vi "FPGARPM.vi"() -> (1 "RPM1 Period (ms)":u32)   [LabVIEW 2019]
uses:
  <vilib>/rvi/Emulation/niFpgaGetClockAttributes.vi
  <vilib>/rvi/Emulation/niFpgaSctlEmulationGetInTimedLoop.vi
  <vilib>/rvi/Emulation/niFpgaEmulationReportErrorSimple.vi
  <vilib>/rvi/eio/common/nirviEmuTemplateMethod_errors.vi
  <vilib>/rvi/Emulation/niFpgaCriticalErrorInLSC.vi
  <vilib>/eio/EIONode/EIONode.xnode
panel:
  out "RPM2 Period (ms)":i16
  # "READ Rotational Speed"
  # "AM Series Inductive Proximity Sensors"
  # "AM1-A0-4H"
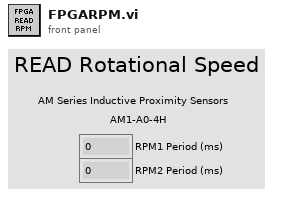
[diagram p1: front panel]
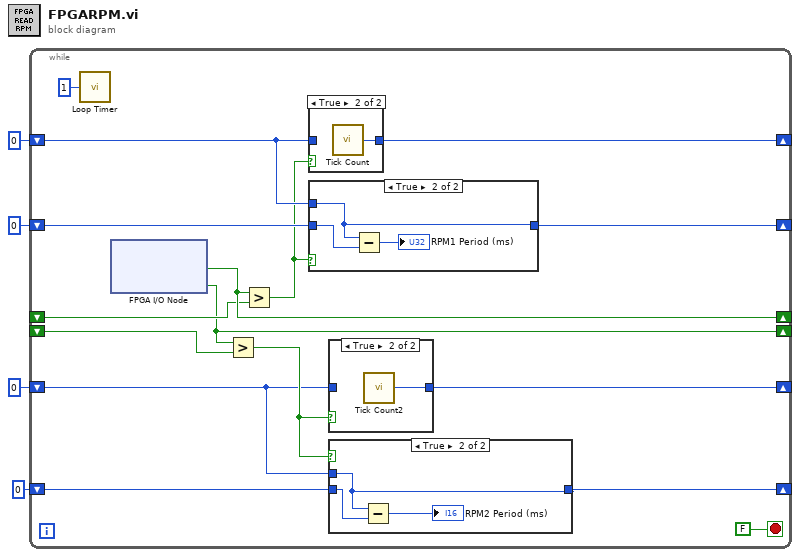
[diagram p0: block diagram]
diagram:
  n1 = while {
    shift-right: [w19] -> _
    shift-left: u32 0 ("Tick Count(Ticks)") -> [w18]
    shift-right: [w16] -> _
    shift-left: u32 0 ("Tick Count(Ticks)") -> [w17]
    shift-right: [w14] -> _
    shift-left: _ -> [w13]
    shift-right: [w12] -> _
    shift-left: i16 0 -> [w8]
    shift-right: [w11] -> _
    shift-left: _ -> [w10]
    shift-right: [w7] -> _
    shift-left: u32 0 ("Tick Count(mSec)") -> [w6]
    stop <- FALSE stop-if-true
    n2 = call "Loop Timer"("Count(mSec)"=u32 1) -> ()  [unwired: 1 out]
    n3 = xnode "FPGA I/O Node"() -> ("Mod2/DI0"=w14:bool, "Mod2/DI1"=w11:bool)  [unwired: 2 in, 2 out]
    n4 = Greater?(x=w11, y=w10) -> (0:w9:bool)
    n5 = Greater?(x=w14, y=w13) -> (0:w15:bool)
    n6 = case shown="True" w15 {
      tunnel: [w31 w32] -> w19
      tunnel: w18 -> [w31 _]
      frame False {
      }
      frame True {
        n7 = call "Tick Count"() -> ("Tick Count(mSec)"=w32:u32)
      }
    }
    n8 = case shown="True" w15 {
      tunnel: w18 -> [_ w30]
      tunnel: [w27 w30] -> w16
      tunnel: w17 -> [w27 w29]
      frame False {
      }
      frame True {
        n9 = Subtract(x=w30, y=w29) -> (x-y=→"RPM1 Period (ms)":u32)
      }
    }
    n10 = case shown="True" w9 {
      tunnel: [w25 w26] -> w12
      tunnel: w8 -> [w25 _]
      frame False {
      }
      frame True {
        n11 = call "Tick Count2"() -> ("Tick Count(mSec)"=w26:u32)
      }
    }
    n12 = case shown="True" w9 {
      tunnel: w8 -> [_ w23]
      tunnel: [w21 w23] -> w7
      tunnel: w6 -> [w21 w22]
      frame False {
      }
      frame True {
        n13 = Subtract(x=w23, y=w22) -> (x-y=→"RPM2 Period (ms)":u32)
      }
    }
  }
